vi "VLC - Script Run (DOTNET).vi"(5 "Script":string, 11 "error in (no error)":errorcluster) -> (6 "VLC Process":refnum<k24>, 15 "error out":errorcluster)   [LabVIEW 2009]
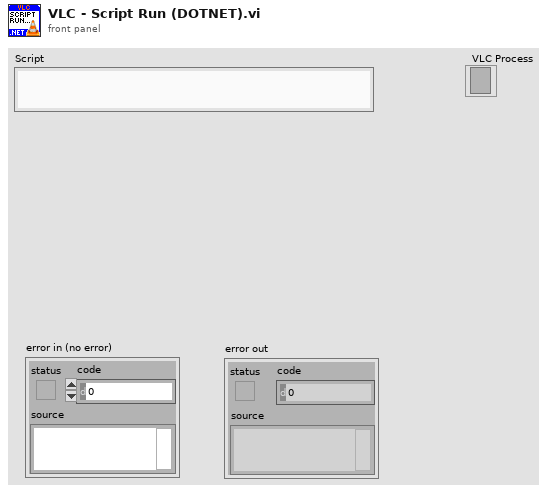
[diagram p1: front panel]
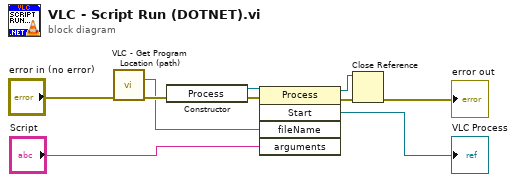
[diagram p0: block diagram]
diagram:
  n1 = call "VLC - Get Program Location (path).vi"("error in (no error)"="error in (no error)") -> ("VLC path"=w6:string, "error out"=w7:errorcluster)  [unwired: 13 in]
  n2 = constructor class="Process"(error in=w7) -> (reference out=w10:refnum<k24>, error out=w9:errorcluster)  [unwired: 2 in, 1 out]
  n3 = invoke class="Process" method="Start"(reference=w10, error in=w9, "fileName"=w6, "arguments"="Script") -> (reference out=w4:refnum<k24>, error out=w5:errorcluster, "Start"=→"VLC Process":refnum<k24>)  [unwired: 1 in, 2 out]
  n4 = Close Reference(reference=w4, error in (no error)=w5) -> (error out=→"error out":errorcluster)
